vi "read_db.vi"(8 "error in (no error)":errorcluster, 10 "Small?":bool, 11 "Constraints":T4 {"Estimate Quality" scale=0.0..5.0; "Lower Mass Limit (kg)" min=-1.0 max=1.0 step=1e-20; "Upper Mass Limit (kg)" min=-1.0 max=1.0 step=1e-20; "Lower Velocity Limit (km/s)" min=-1.0 max=299792000.0; "Upper Velocity Limit (km/s)" min=-1.0 max=299792000.0}) -> (0 "error out":errorcluster, 1 "Experiment Settings ID Array":i64[](array[numeric]), 2 "Dust Event ID Array":i64[](array[numeric]), 3 "Dust Array":T1[](array[typedef]) {"File Location" items=["Unknown"=-1, "Processing"=0, "Storage"=1]; "Estimate Source" items=["Any Source."=-2, "No Shot"=-1, "Basic Labview Estimate"=0, "IDL Estimate From Andrew"=1, "IDL Estimate From Tobin"=2, "Old Metadata"=3]}, 5 "File Location Array":i64[](array[numeric]))   [LabVIEW 2013]
uses:
  Controls/Constraints.ctl
  Public API/Query_Dust_Event.ctl
  Controls/Estimate_source.ctl
  Controls/File_location.ctl
  <vilib>/addons/database/Auxilliary.llb/DB Tools Cursor Type.ctl
  <userlib>/_OpenG.lib/array/array.llb/Remove Duplicates from 1D Array (String)__ogtk.vi
  <userlib>/_OpenG.lib/array/array.llb/Search 1D Array (String)__ogtk.vi
  <userlib>/_OpenG.lib/array/array.llb/Delete Elements from 1D Array (String)__ogtk.vi
  <vilib>/addons/database/Connection.llb/Conn Execute.vi
  <vilib>/addons/database/Recordset.llb/Rec Fetch Recordset Data (R).vi
  <vilib>/addons/database/Recordset.llb/Rec Destroy - Connection.vi
  <vilib>/addons/database/_DB Variant To Data/Database Variant To Data.xnode
  <vilib>/addons/database/NI_Database_API.lvlib
panel:
  out "SQL Query Sintax":string
  # "Dust Event"
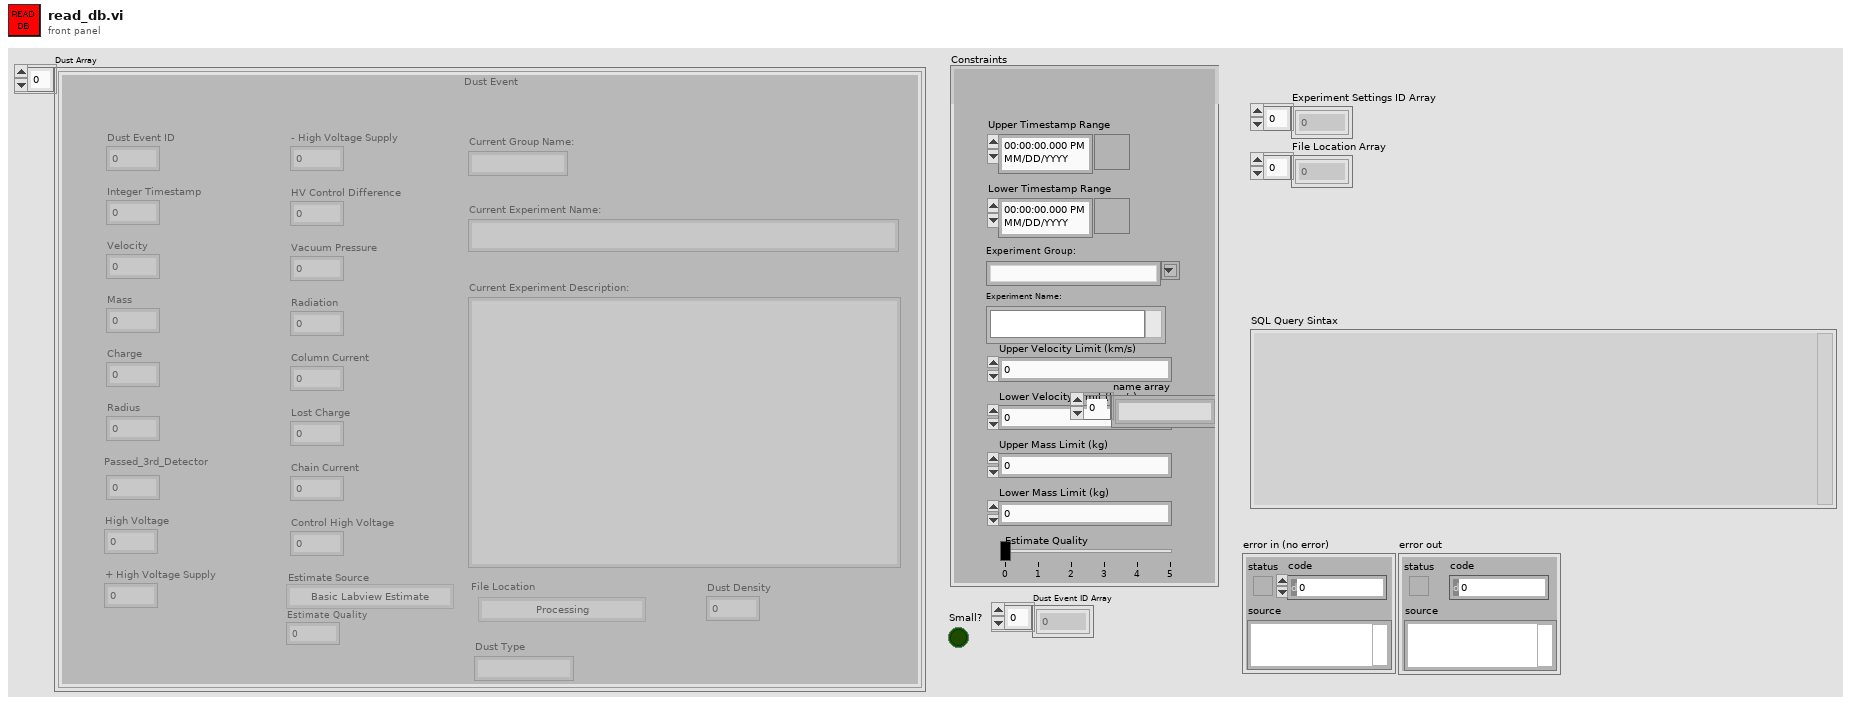
[diagram p1: front panel]
types:
  T1 = typedef "Query_Dust_Event.ctl" = cluster{"Dust Event ID":i64, "Integer Timestamp":i64, "Velocity":sgl, "Mass":sgl, "Charge":sgl, "Radius":sgl, "Passed_3rd_Detector":i8, "High Voltage":sgl, "+ High Voltage Supply":sgl, "- High Voltage Supply":sgl, "HV Control Difference":sgl, "Vacuum Pressure":sgl, "Radiation":sgl, "Column Current":sgl, "Lost Charge":sgl, "Chain Current":sgl, "Control High Voltage":sgl, "Current Group Name:":string, "Current Experiment Name:":string, "Current Experiment Description:":string, "Estimate Source":T2, "Estimate Quality":sgl, "File Location":T3, "Dust Type":string, "Dust Density":sgl}
  T2 = typedef "Estimate_source.ctl" = i8
  T3 = typedef "File_location.ctl" = i8
  T4 = typedef "Constraints.ctl" = cluster{"Upper Timestamp Range":timestamp, "Lower Timestamp Range":timestamp, "Experiment Group:":string, "Experiment Name:":i32[], "Upper Velocity Limit (km/s)":dbl, "Lower Velocity Limit (km/s)":dbl, "Upper Mass Limit (kg)":dbl, "Lower Mass Limit (kg)":dbl, "name array":string[], "Estimate Quality":cluster{dbl, dbl}}
  T5 = typedef "NI_Database_API.lvlib/DB Tools Cursor Type.ctl" = enum16{"forward-only", "keyset", "dynamic", "static"}
  T6 = typedef "NI_Database_API.lvlib/Conn ObjectReference.ctl" = refnum<k1>
  T7 = typedef "NI_Database_API.lvlib/Rec ObjectReference.ctl" = refnum<k1>
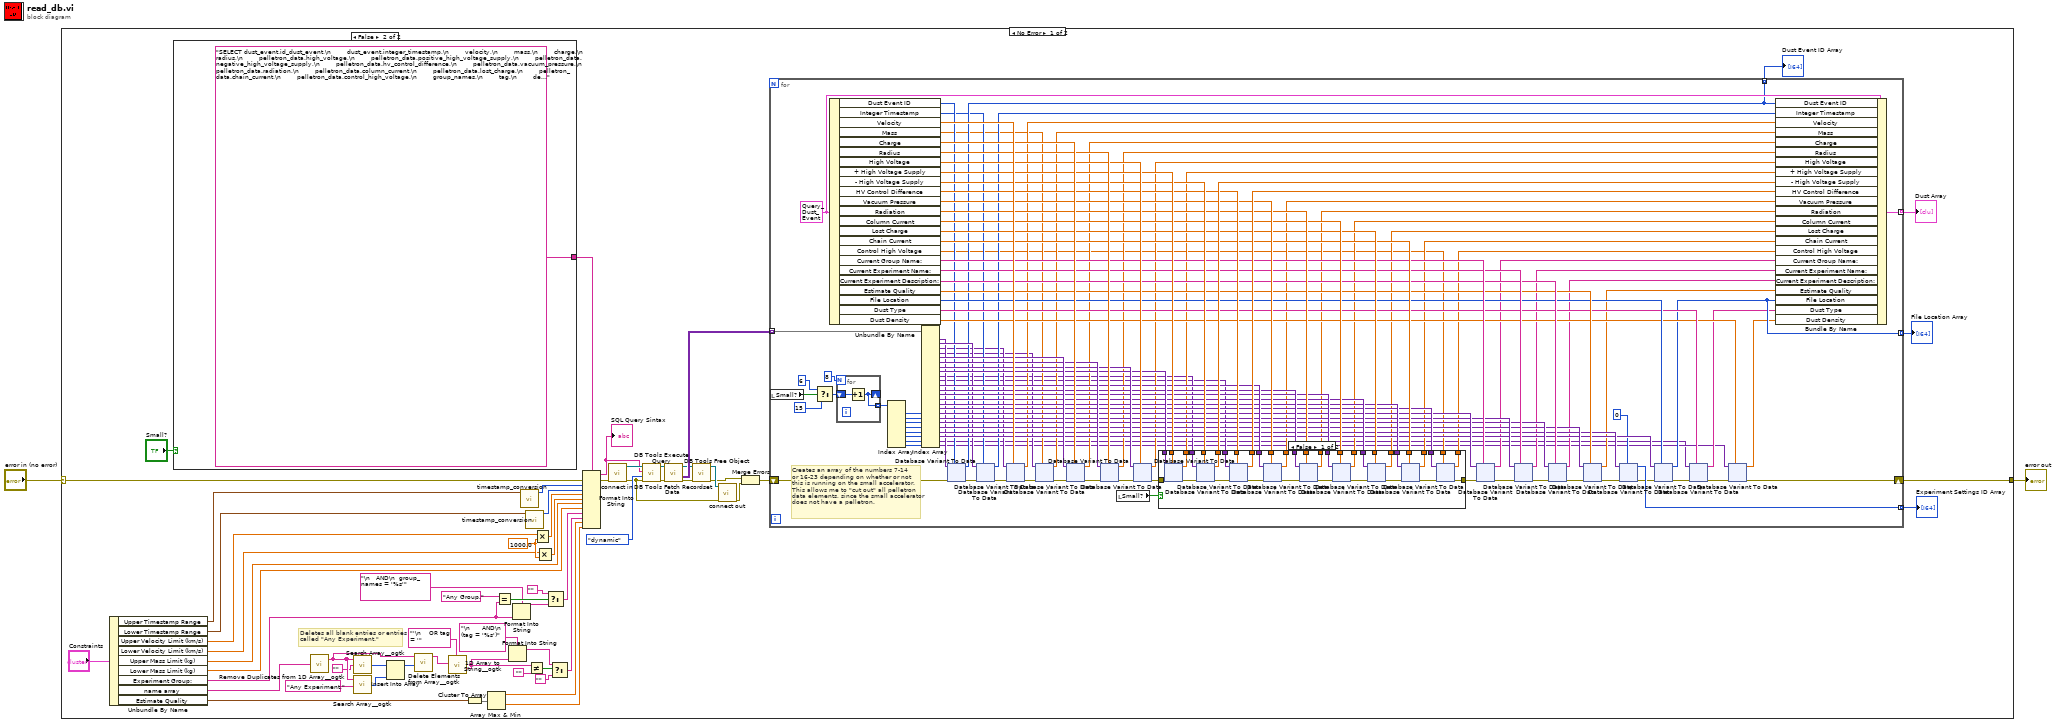
[diagram p0: block diagram]
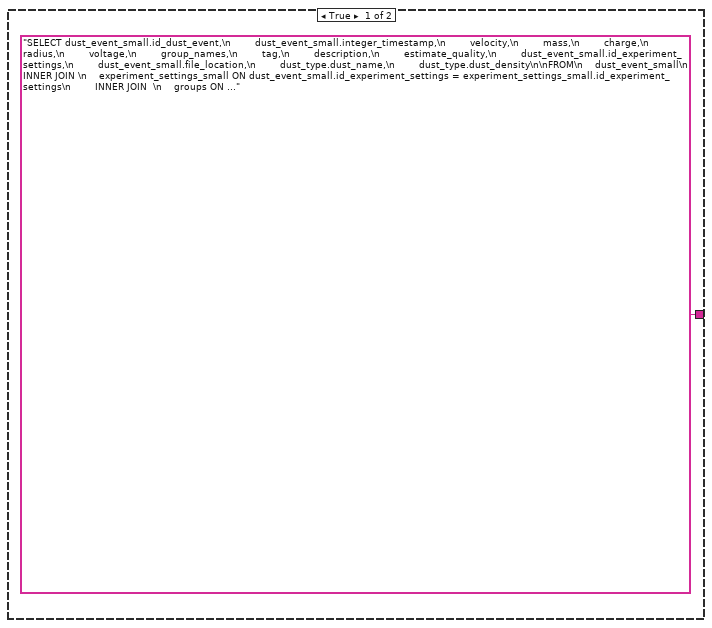
[diagram p2: hidden frame]
diagram:
  n1 = case shown="No Error" "error in (no error)" {
    selector: "error in (no error)" -> [w36 w990]
    tunnel: [w37 w990] -> w1
    frame No Error {
      w47 = 1000.0 ("y")
      # "Deletes all blank entries or entries\ncalled \"Any Experiment.\""
      n2 = Unbundle By Name("Constraints") -> ("Upper Timestamp Range"=w14:timestamp, "Lower Timestamp Range"=w13:timestamp, "Upper Velocity Limit (km/s)"=w9:dbl, "Lower Velocity Limit (km/s)"=w10:dbl, "Upper Mass Limit (kg)"=w11:dbl, "Lower Mass Limit (kg)"=w12:dbl, "Experiment Group:"=w6:string, "name array"=w15:string[], "Estimate Quality"=w46:cluster{dbl, dbl})
      n3 = case shown="False" "Small?" {
        tunnel: ["SELECT dust_event_small.id_dust_event,\n        dust_event_small.integer_timestamp,\n        velocity,\n        mass,\n        charge,\n        radius,\n        voltage,\n        group_names,\n        tag,\n        description,\n        estimate_quality,\n        dust_event_small.id_experiment_settings,\n        dust_event_small.file_location,\n        dust_type.dust_name,\n        dust_type.dust_density\n\nFROM\n    dust_event_small\n        INNER JOIN \n    experiment_settings_small ON dust_event_small.id_experiment_settings = experiment_settings_small.id_experiment_settings\n        INNER JOIN  \n    groups ON experiment_settings_small.id_groups=groups.id_groups\n        INNER JOIN\n    dust_info_small ON dust_event_small.id_dust_info = dust_info_small.id_dust_info\n      \t\tINNER JOIN\n   \tdust_type ON dust_info_small.dust_type = dust_type.id_dust_type\n\nWHERE\n  dust_event_small.integer_timestamp <= %d AND dust_event_small.integer_timestamp >= %d\n    AND\n  dust_event_small.velocity <= %d AND dust_event_small.velocity >= %d\n    AND\n  dust_event_small.mass <= %d AND dust_event_small.mass >= %d%s%s\n    AND\n  dust_event_small.estimate_quality <= %d AND dust_event_small.estimate_quality >= %d\nORDER BY\n  dust_event_small.id_dust_event; " ("string") "SELECT dust_event.id_dust_event,\n        dust_event.integer_timestamp,\n        velocity,\n        mass,\n        charge,\n        radius,\n        pelletron_data.high_voltage,\n        pelletron_data.positive_high_voltage_supply,\n        pelletron_data.negative_high_voltage_supply,\n        pelletron_data.hv_control_difference,\n        pelletron_data.vacuum_pressure,\n        pelletron_data.radiation,\n        pelletron_data.column_current,\n        pelletron_data.lost_charge,\n        pelletron_data.chain_current,\n        pelletron_data.control_high_voltage,\n        group_names,\n        tag,\n        description,\n        estimate_quality,\n        dust_event.id_experiment_settings,\n        dust_event.file_location,\n        dust_type.dust_name,\n        dust_type.dust_density\n\nFROM\n    dust_event\n        INNER JOIN \n    experiment_settings ON dust_event.id_experiment_settings = experiment_settings.id_experiment_settings\n        INNER JOIN  \n    groups ON experiment_settings.id_groups=groups.id_groups\n        INNER JOIN\n    pelletron_data ON pelletron_data.id_pelletron_data = dust_event.id_pelletron_data\nINNER JOIN\n     dust_info ON dust_event.id_dust_info = dust_info.id_dust_info\n\t\tINNER join\n\tdust_type ON dust_info.dust_type = dust_type.id_dust_type\n\nWHERE\n  dust_event.integer_timestamp <= %d  AND dust_event.integer_timestamp >= %d\n    AND\n  dust_event.velocity <= %d  AND dust_event.velocity >= %d\n    AND\n  dust_event.mass <= %d  AND dust_event.mass >= %d%s%s\n    AND\n  dust_event.estimate_quality <= %d AND dust_event.estimate_quality >= %d\nORDER BY\n  dust_event.id_dust_event; " ("string")] -> w49
        frame True {
        }
        frame False {
        }
      }
      n4 = call-poly <userlib>:"Remove Duplicates from 1D Array__ogtk.vi"("Input Array"=w15) -> ("Output Array"=w28:string[])  [unwired: 1 out]
      n5 = call-poly <userlib>:"Search Array__ogtk.vi"("Array"=w28, "Element Data"="") -> ("Indices of Elements"=w23:i32[])  [unwired: 7 in]
      n6 = call-poly <userlib>:"Search Array__ogtk.vi"("Array"=w28, "Element Data"="Any Experiment.") -> ("Indices of Elements"=w30:i32[])  [unwired: 7 in]
      n7 = Insert Into Array(array=w23, new element=w30) -> (w29:i32[])  [unwired: 1 in]
      n8 = call-poly <userlib>:"Delete Elements from Array__ogtk.vi"("indices"=w29, "array"=w28) -> ("array w/ subset deleted"=w24:string[])  [unwired: 8 in, 1 out]
      n9 = call <userlib>:"1D Array to String__ogtk.vi"("delimiter (Tab)"="'\n    OR tag = '", "Array of Strings"=w24) -> ("delimited string"=w26:string)  [unwired: 9 in]
      n10 = Cluster To Array(cluster=w46) -> (array=w45:dbl[])
      n11 = Array Max & Min(array=w45) -> (max value=w19:dbl, min value=w18:dbl)  [unwired: 2 out]
      n12 = Equal?(x="Any Group.", y=w6) -> (x = y?=w60:bool)
      n13 = Format Into String(format string="\n      AND\n    (tag = '%s')" ("string"), w26) -> (resulting string=w32:string)  [unwired: 2 in, 1 out]
      n14 = Format Into String(format string="\n   AND\n  group_names = '%s'" ("string"), w6) -> (resulting string=w38:string)  [unwired: 2 in, 1 out]
      n15 = call "timestamp_conversion.vi"("Time Stamp"=w14) -> ("Integer Time"=w51:i64)  [unwired: 8 in, 1 out]
      n16 = call "timestamp_conversion.vi"("Time Stamp"=w13) -> ("Integer Time"=w50:i64)  [unwired: 8 in, 1 out]
      n17 = Not Equal?(x=w26, y="") -> (x != y?=w31:bool)
      n18 = Multiply(x=w9, y=w47) -> (x*y=w8:dbl)
      n19 = Multiply(x=w10, y=w47) -> (x*y=w7:dbl)
      n20 = Select(t="", s=w60, f=w38) -> (s? t:f=w17:string)
      n21 = Select(t=w32, s=w31, f="") -> (s? t:f=w16:string)
      n22 = Format Into String(format string=w49, error in=w36, w51, w50, w8, w7, w11, w12, w17, w16, w19, w18) -> (resulting string=w39:string, error out=w34:errorcluster)  [unwired: 1 in]
      "SQL Query Sintax" <- w39
      n23 = call "connect in.vi"("error in (no error)"=w34) -> ("error out"=w3:errorcluster, "Database Connection"=w61:T6)  [unwired: 6 in, 1 out]
      n24 = call-poly <vilib>:"DB Tools Execute Query.vi"("error in (no error)"=w3, "cursor type"=DB_Tools_Cursor_Type."dynamic", "SQL query"=w39, "connection reference"=w61) -> ("error out"=w62:errorcluster, "recordset reference"=w63:T7)  [unwired: 4 in]
      n25 = call-poly <vilib>:"DB Tools Fetch Recordset Data.vi"("error in (no error)"=w62, "recordset reference"=w63) -> ("error out"=w43:errorcluster, "recordset data"=w58:variant[][], "recordset reference out"=w42:T7)  [unwired: 3 in]
      n26 = call-poly <vilib>:"DB Tools Free Object.vi"("error in (no error)"=w43, "recordset reference"=w42) -> ("error out"=w4:errorcluster, "connection reference"=w40:T6)  [unwired: 8 in]
      n27 = call "connect out.vi"("error in (no error)"=w3, "connection reference"=w40) -> ("error out"=w41:errorcluster)  [unwired: 9 in]
      n28 = Merge Errors(w4, w41) -> (w5:errorcluster)
      n29 = for {
        tunnel: w58 -> [w172] mode=indexing
        shift-right: [w132] -> w37
        shift-left: w5 -> [w171]
        tunnel: [w142] -> w57 mode=indexing
        tunnel: [w111] -> w54 mode=indexing
        tunnel: [w139] -> w53 mode=indexing
        tunnel: [w85] -> w48 mode=indexing
        w170 = T1 {"Dust Event ID"=0, "Integer Timestamp"=0, "Velocity"=0.0, "Mass"=0.0, "Charge"=0.0, "Radius"=0.0, "Passed_3rd_Detector"=0, "High Voltage"=0.0, "+ High Voltage Supply"=0.0, "- High Voltage Supply"=0.0, "HV Control Difference"=0.0, "Vacuum Pressure"=0.0, "Radiation"=0.0, "Column Current"=0.0, "Lost Charge"=0.0, "Chain Current"=0.0, "Control High Voltage"=0.0, "Current Group Name:"="", "Current Experiment Name:"="", "Current Experiment Description:"="", "Estimate Source"=0, "Estimate Quality"=0.0, "File Location"=0, "Dust Type"="", "Dust Density"=0.0} ("Cluster")
        # "Creates an array of the numbers 7-14\nor 16-23 depending on whether or not\nthis is running on the small accelerator.\nThis allows me to \"cut out\" all pelletron\ndata elements, since the small accelerator\ndoes not have a pelletron."
        n30 = local read "Small?"() -> (w68:bool)
        n31 = Select(t=6 ("index"), s=w68, f=15) -> (s? t:f=w70:i32)
        n32 = Unbundle By Name(w170) -> ("Dust Event ID"=w112:i64, "Integer Timestamp"=w110:i64, "Velocity"=w168:sgl, "Mass"=w105:sgl, "Charge"=w165:sgl, "Radius"=w161:sgl, "High Voltage"=w159:sgl, "+ High Voltage Supply"=w157:sgl, "- High Voltage Supply"=w156:sgl, "HV Control Difference"=w154:sgl, "Vacuum Pressure"=w152:sgl, "Radiation"=w151:sgl, "Column Current"=w150:sgl, "Lost Charge"=w149:sgl, "Chain Current"=w148:sgl, "Control High Voltage"=w92:sgl, "Current Group Name:"=w146:string, "Current Experiment Name:"=w144:string, "Current Experiment Description:"=w143:string, "Estimate Quality"=w141:sgl, "File Location"=w137:T3, "Dust Type"=w135:string, "Dust Density"=w134:sgl)
        n33 = for {
          N: 8 -> [_]
          shift-right: [w173] -> _
          shift-left: w70 -> [w174]
          tunnel: [w173] -> w80 mode=indexing
          n34 = Increment(x=w174) -> (x+1=w173:i32)
        }
        n35 = Index Array(array=w80) -> (element #1=w78:i32, element #2=w77:i32, element #3=w76:i32, element #4=w75:i32, element #5=w74:i32, element #6=w73:i32, element #7=w72:i32, element #8=w71:i32)  [unwired: 8 in]
        n36 = Index Array(array=w172, index #17=w78, index #18=w77, index #19=w76, index #20=w75, index #21=w74, index #22=w73, index #23=w72, index #24=w71) -> (element #1=w113:variant, element #2=w114:variant, element #3=w108:variant, element #4=w106:variant, element #5=w164:variant, element #6=w160:variant, element #7=w128:variant, element #8=w127:variant, element #9=w99:variant, element #10=w98:variant, element #11=w126:variant, element #12=w125:variant, element #13=w124:variant, element #14=w123:variant, element #15=w122:variant, element #16=w121:variant, element #17=w120:variant, element #18=w119:variant, element #19=w118:variant, element #20=w117:variant, element #21=w116:variant, element #22=w115:variant, element #23=w81:variant, element #24=w82:variant)  [unwired: 16 in]
        n37 = xnode "Database Variant To Data"("database variant"=w113, "error in"=w171, "type"=w112) -> ("data"=w111:i64, "error out"=w169:errorcluster)
        n38 = xnode "Database Variant To Data"("database variant"=w114, "error in"=w169, "type"=w110) -> ("data"=w109:i64, "error out"=w167:errorcluster)
        n39 = xnode "Database Variant To Data"("database variant"=w108, "error in"=w167, "type"=w168) -> ("data"=w107:sgl, "error out"=w166:errorcluster)
        n40 = xnode "Database Variant To Data"("database variant"=w106, "error in"=w166, "type"=w105) -> ("data"=w104:sgl, "error out"=w163:errorcluster)
        n41 = xnode "Database Variant To Data"("database variant"=w164, "error in"=w163, "type"=w165) -> ("data"=w103:sgl, "error out"=w162:errorcluster)
        n42 = xnode "Database Variant To Data"("database variant"=w160, "error in"=w162, "type"=w161) -> ("data"=w102:sgl, "error out"=w129:errorcluster)
        n43 = local read "Small?"() -> (w66:bool)
        n44 = xnode "Database Variant To Data"("database variant"=w128, "error in"=w129, "type"=w159) -> ("data"=w101:sgl, "error out"=w158:errorcluster)
        n45 = case shown="False" w66 {
          tunnel: w158 -> [w211 w500]
          tunnel: w157 -> [w210 w509]
          tunnel: w156 -> [w209 w508]
          tunnel: [w208 w508] -> w155
          tunnel: w154 -> [w205 w507]
          tunnel: [w204 w507] -> w153
          tunnel: w152 -> [w202 w506]
          tunnel: w151 -> [w200 w505]
          tunnel: w150 -> [w198 w504]
          tunnel: w149 -> [w196 w503]
          tunnel: w148 -> [w194 w502]
          tunnel: [w192 w500] -> w147
          tunnel: w127 -> [w191 _]
          tunnel: w126 -> [w190 _]
          tunnel: w125 -> [w189 _]
          tunnel: w124 -> [w188 _]
          tunnel: w123 -> [w187 _]
          tunnel: w122 -> [w186 _]
          tunnel: w121 -> [w185 _]
          tunnel: [w184 w509] -> w100
          tunnel: w99 -> [w183 _]
          tunnel: w98 -> [w182 _]
          tunnel: [w181 w506] -> w97
          tunnel: [w180 w505] -> w96
          tunnel: [w179 w504] -> w95
          tunnel: [w178 w503] -> w94
          tunnel: [w177 w502] -> w93
          tunnel: w92 -> [w176 w501]
          tunnel: [w175 w501] -> w91
          frame False {
            n46 = xnode "Database Variant To Data"("database variant"=w191, "error in"=w211, "type"=w210) -> ("data"=w184:sgl, "error out"=w207:errorcluster)
            n47 = xnode "Database Variant To Data"("database variant"=w183, "error in"=w207, "type"=w209) -> ("data"=w208:sgl, "error out"=w206:errorcluster)
            n48 = xnode "Database Variant To Data"("database variant"=w182, "error in"=w206, "type"=w205) -> ("data"=w204:sgl, "error out"=w203:errorcluster)
            n49 = xnode "Database Variant To Data"("database variant"=w190, "error in"=w203, "type"=w202) -> ("data"=w181:sgl, "error out"=w201:errorcluster)
            n50 = xnode "Database Variant To Data"("database variant"=w189, "error in"=w201, "type"=w200) -> ("data"=w180:sgl, "error out"=w199:errorcluster)
            n51 = xnode "Database Variant To Data"("database variant"=w188, "error in"=w199, "type"=w198) -> ("data"=w179:sgl, "error out"=w197:errorcluster)
            n52 = xnode "Database Variant To Data"("database variant"=w187, "error in"=w197, "type"=w196) -> ("data"=w178:sgl, "error out"=w195:errorcluster)
            n53 = xnode "Database Variant To Data"("database variant"=w186, "error in"=w195, "type"=w194) -> ("data"=w177:sgl, "error out"=w193:errorcluster)
            n54 = xnode "Database Variant To Data"("database variant"=w185, "error in"=w193, "type"=w176) -> ("data"=w175:sgl, "error out"=w192:errorcluster)
          }
          frame True {
          }
        }
        n55 = xnode "Database Variant To Data"("database variant"=w120, "error in"=w147, "type"=w146) -> ("data"=w90:string, "error out"=w145:errorcluster)
        n56 = xnode "Database Variant To Data"("database variant"=w119, "error in"=w145, "type"=w144) -> ("data"=w89:string, "error out"=w130:errorcluster)
        n57 = xnode "Database Variant To Data"("database variant"=w118, "error in"=w130, "type"=w143) -> ("data"=w88:string, "error out"=w131:errorcluster)
        n58 = xnode "Database Variant To Data"("database variant"=w117, "error in"=w131, "type"=w141) -> ("data"=w87:sgl, "error out"=w140:errorcluster)
        n59 = xnode "Database Variant To Data"("database variant"=w116, "error in (no error)"=w140, "type"=i64 0 ("Dust Event ID")) -> ("data"=w139:i64, "error out"=w138:errorcluster)
        n60 = xnode "Database Variant To Data"("database variant"=w115, "error in (no error)"=w138, "type"=w137) -> ("data"=w85:T3, "error out"=w133:errorcluster)
        n61 = xnode "Database Variant To Data"("database variant"=w81, "error in"=w133, "type"=w135) -> ("data"=w84:string, "error out"=w136:errorcluster)
        n62 = xnode "Database Variant To Data"("database variant"=w82, "error in"=w136, "type"=w134) -> ("data"=w83:sgl, "error out"=w132:errorcluster)
        n63 = Bundle By Name(cluster=w170, "Dust Event ID"=w111, "Integer Timestamp"=w109, "Velocity"=w107, "Mass"=w104, "Charge"=w103, "Radius"=w102, "High Voltage"=w101, "+ High Voltage Supply"=w100, "- High Voltage Supply"=w155, "HV Control Difference"=w153, "Vacuum Pressure"=w97, "Radiation"=w96, "Column Current"=w95, "Lost Charge"=w94, "Chain Current"=w93, "Control High Voltage"=w91, "Current Group Name:"=w90, "Current Experiment Name:"=w89, "Current Experiment Description:"=w88, "Estimate Quality"=w87, "File Location"=w85, "Dust Type"=w84, "Dust Density"=w83) -> (w142:T1)
      }
      "Dust Array" <- w57
      "Dust Event ID Array" <- w54
      "Experiment Settings ID Array" <- w53
      "File Location Array" <- w48
    }
    frame Error {
    }
  }
  "error out" <- w1
